vi "Set Output.vi"(8 "error":errorcluster, 9 "Settle (0 mS)":u32, 10 "Output ON":bool, 11 "VISA in":refnum<visa-resource-name>) -> (0 "error out":errorcluster, 3 "VISA out":refnum<visa-resource-name>)   [LabVIEW 2023, in "TDK20-38 API.lvlib"]
uses:
  TDK20-38 API.lvlib
  <userlib>/TDK-Lambda GEN LAN Series/TDK-Lambda GEN LAN Series.lvlib
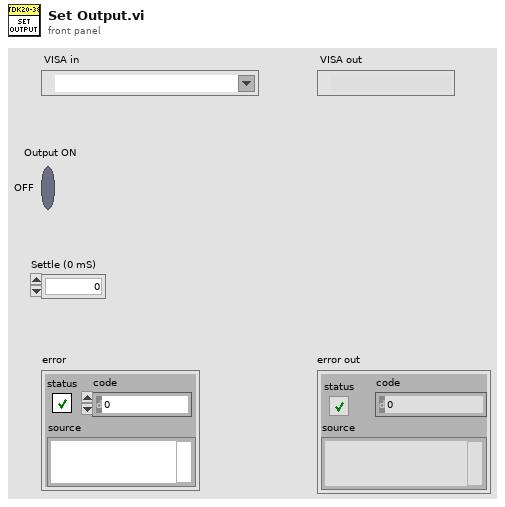
[diagram p1: front panel]
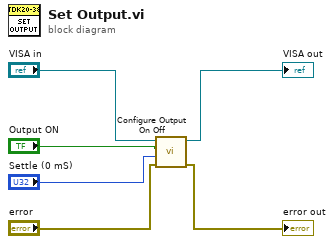
[diagram p0: block diagram]
diagram:
  n1 = call <userlib>:"Configure Output On Off.vi"("error"="error", "Settle (0 mS)"="Settle (0 mS)", "Output ON"="Output ON", "VISA"="VISA in") -> ("error out"=→"error out":errorcluster, "VISA out"=→"VISA out":refnum<visa-resource-name>)  [unwired: 6 in]
